vi "Configure Data Width.vi"(8 "error in (no error)":errorcluster, 11 "VISA resource name":refnum<visa-resource-name>) -> (0 "error out":errorcluster, 2 "Width":i32, 3 "VISA resource name out":refnum<visa-resource-name>)   [LabVIEW 2011]
doc: "Configures the data width of the oscilloscope."
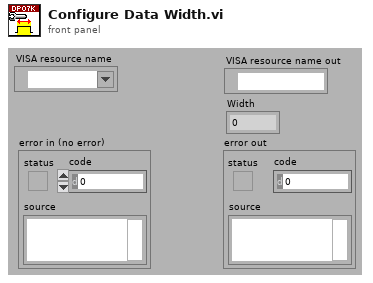
[diagram p1: front panel]
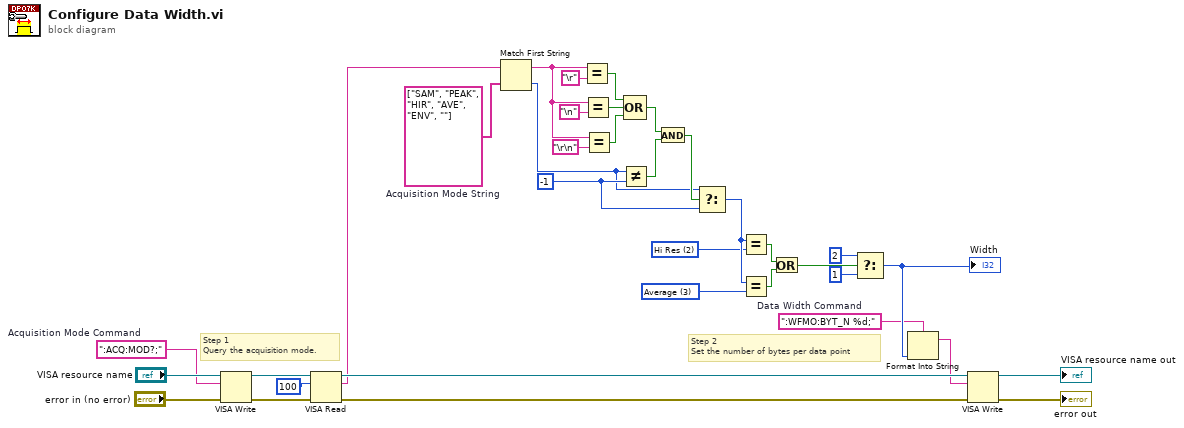
[diagram p0: block diagram]
diagram:
  w2 = u16 3 items=["Sample", "Peak Detect", "Hi Res", "Average", "Envelope"] ("Acquisition Mode (0:Sample)")
  w3 = u16 2 items=["Sample", "Peak Detect", "Hi Res", "Average", "WfmDB", "Envelope"] ("Acquisition Mode (0:Sample)")
  w26 = -1 ("y")
  w12 = ":WFMO:BYT_N %d;"  # Data Width Command
  w14 = string[] ["SAM", "PEAK", "HIR", "AVE", "ENV", ""]  # Acquisition Mode String
  w4 = ":ACQ:MOD?;"  # Acquisition Mode Command
  # "Step 2       \nSet the number of bytes per data point"
  # "Step 1       \nQuery the acquisition mode."
  n1 = VISA Write(VISA resource name="VISA resource name", write buffer=w4, error in (no error)="error in (no error)") -> (VISA resource name out=w5:refnum<visa-resource-name>, error out=w6:errorcluster)  [unwired: 1 out]
  n2 = VISA Read(VISA resource name=w5, byte count=u32 100, error in (no error)=w6) -> (VISA resource name out=w32:refnum<visa-resource-name>, read buffer=w15:string, error out=w35:errorcluster)  [unwired: 1 out]
  n3 = Match First String(2:w14, 3:w15) -> (0:w25:i32, 1:w19:string)
  n4 = Equal?(x=w19, y="\r" ("Carriage Return Constant")) -> (x = y?=w20:bool)
  n5 = Equal?(x=w19, y="\n" ("Line Feed Constant")) -> (x = y?=w21:bool)
  n6 = Equal?(x=w19, y="\r\n" ("End of Line Constant")) -> (x = y?=w22:bool)
  n7 = Not Equal?(x=w25, y=w26) -> (x != y?=w24:bool)
  n8 = Compound Arithmetic op=OR(w20, w21, w22) -> (w23:bool)
  n9 = And(x=w23, y=w24) -> (x .and. y?=w27:bool)
  n10 = Select(t=w25, s=w27, f=w26) -> (s? t:f=w28:i32)
  n11 = Equal?(x=w28, y=w3) -> (x = y?=w8:bool)
  n12 = Equal?(x=w28, y=w2) -> (x = y?=w9:bool)
  n13 = Or(x=w8, y=w9) -> (x .or. y?=w29:bool)
  n14 = Select(t=2 ("f"), s=w29, f=1) -> (s? t:f=w13:i32)
  "Width" <- w13
  n15 = Format Into String(format string=w12, w13) -> (resulting string=w1:string)  [unwired: 2 in, 1 out]
  n16 = VISA Write(VISA resource name=w32, write buffer=w1, error in (no error)=w35) -> (VISA resource name out=→"VISA resource name out":refnum<visa-resource-name>, error out=→"error out":errorcluster)  [unwired: 1 out]
